vi "Write MType+MSerial.vi"(5 "MType":string, 7 "MSerial":string, 8 "error in":errorcluster, 11 "XLS in":refnum<class "XLS.lvclass">) -> (0 "error out":errorcluster, 3 "XLS out":refnum<class "XLS.lvclass">)   [LabVIEW 2017, in "Report_lib.lvlib" / "XLS.lvclass"]
uses:
  XLS.lvclass
  XLS.lvclass/XLS.ctl
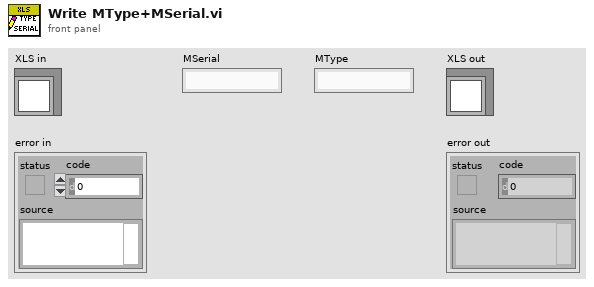
[diagram p1: front panel]
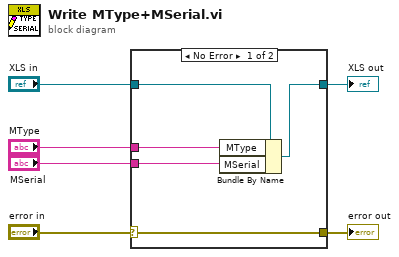
[diagram p0: block diagram]
diagram:
  n1 = case shown="No Error" "error in" {
    selector: "error in" -> [w11 w12]
    tunnel: [w11 w12] -> w5
    tunnel: [w9 w13] -> w3
    tunnel: "XLS in" -> [w10 w13]
    tunnel: "MType" -> [w8 _]
    tunnel: "MSerial" -> [w7 _]
    frame No Error {
      n2 = Bundle By Name(cluster=w10, "MType"=w8, "MSerial"=w7) -> (w9:refnum<class "XLS.lvclass">)
    }
    frame Error {
    }
  }
  "error out" <- w5
  "XLS out" <- w3
